vi "Read SPI Channel (0).vi"(8 "error in (no error)":errorcluster, 11 "LINX SPI in":refnum<class "LINX SPI.lvclass">) -> (0 "error out":errorcluster, 2 "SPI Channel (0)":u8, 3 "LINX SPI out":refnum<class "LINX SPI.lvclass">)   [LabVIEW 2020, in "LINX SPI.lvclass"]
uses:
  LINX SPI.lvclass
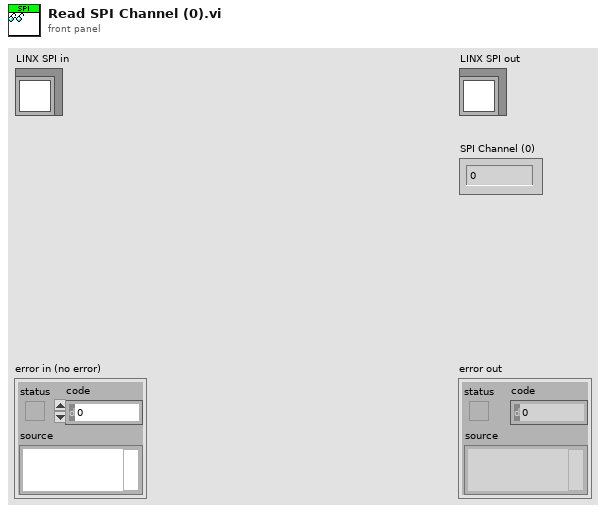
[diagram p1: front panel]
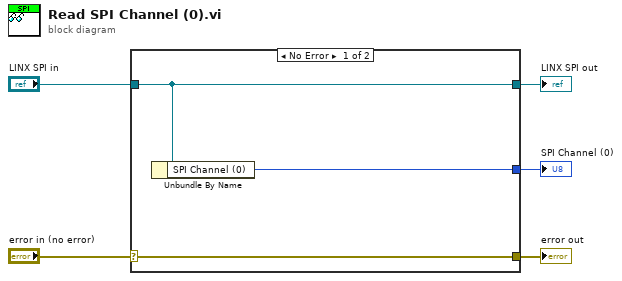
[diagram p0: block diagram]
diagram:
  n1 = case shown="No Error" "error in (no error)" {
    selector: "error in (no error)" -> [w8 w9]
    tunnel: [w8 w9] -> w4
    tunnel: [w7 w10] -> w2
    tunnel: "LINX SPI in" -> [w7 w10]
    tunnel: [w6 _] -> w1
    frame No Error {
      n2 = Unbundle By Name(w7) -> ("SPI Channel (0)"=w6:u8)
    }
    frame Error {
    }
  }
  "error out" <- w4
  "LINX SPI out" <- w2
  "SPI Channel (0)" <- w1
